vi "Main.vi"() -> ()   [LabVIEW 2021]
uses:
  <vilib>/Instr/_visa.llb/VISA Configure Serial Port (Instr).vi
  <extravilib>/ChannelInstances/Event Messenger-str/Instantiate.vi
  <extravilib>/ChannelInstances/Event Messenger-str/))Channel.vi
  <extravilib>/ChannelInstances/Event Messenger-str.lvlib
panel:
  out "Arduino":errorcluster
  in  "Exit":bool
  in  "VISA name":refnum<visa-resource-name>
  out "Ready":bool
  out "Finish":bool
  out "Start":bool
  out "Time":picture
  in  "Ready?":bool
  in  "Reset":bool
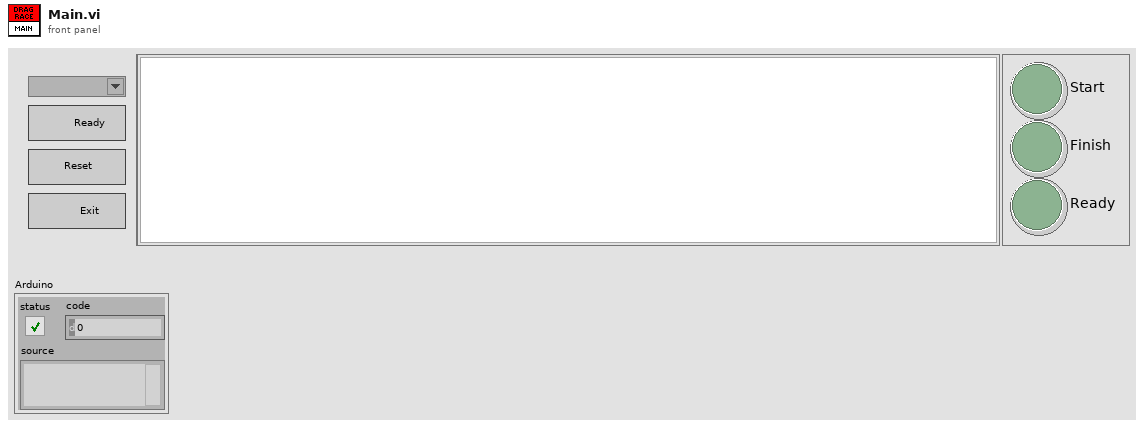
[diagram p1: front panel]
types:
  T1 = enum8{"Enabled", "Disabled", "Disabled and Grayed Out"}
  T2 = typedef "Event Messenger-str.lvlib/))Channel.ctl" = refnum<queue>
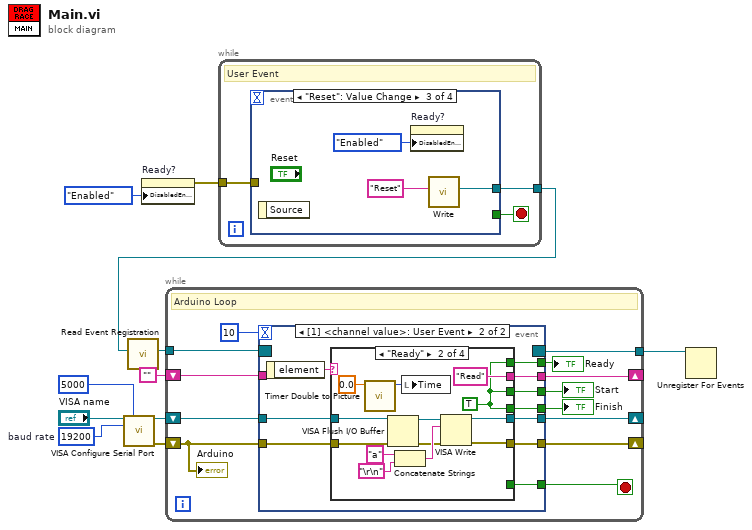
[diagram p0: block diagram]
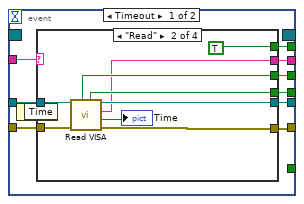
[diagram p2: hidden frame]
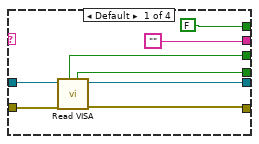
[diagram p3: hidden frame]
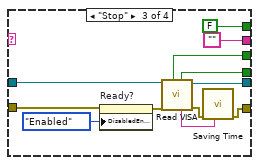
[diagram p4: hidden frame]
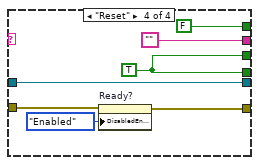
[diagram p5: hidden frame]
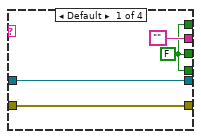
[diagram p6: hidden frame]
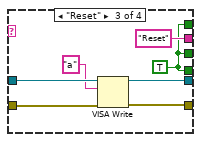
[diagram p7: hidden frame]
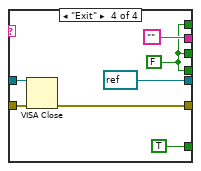
[diagram p8: hidden frame]
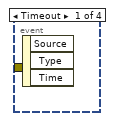
[diagram p9: hidden frame]
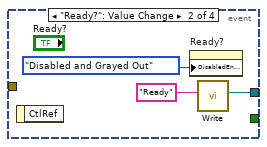
[diagram p10: hidden frame]
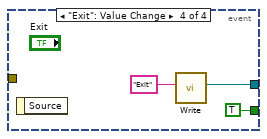
[diagram p11: hidden frame]
diagram:
  w10 = u32 19200  # baud rate
  n1 = call-poly "VISA Configure Serial Port"("VISA resource name"="VISA name", "timeout (10sec)"=u32 5000, "baud rate (9600)"=w10) -> ("VISA resource name out"=w9:refnum<visa-resource-name>, "error out"=w8:errorcluster)  [unwired: 11 in]
  n2 = property on="Ready?" class="Bool"("DisabledEnum"=T1."Enabled" ("Disabled")) -> (error out=w3:errorcluster)  [unwired: 2 in, 1 out]
  n3 = while {
    tunnel: [w14] -> w7
    tunnel: w3 -> [w12]
    stop <- w13 stop-if-true
    # "User Event"
    n4 = event shown="[2] \"Reset\": Value Change" {
      selector: _ -> [_ _ _ _]
      dyn-events: _ -> [_ _ _ _]
      timeout: _ -> [_ _ _ _]
      tunnel: [_ w16 w19 w22] -> w14
      tunnel: [_ _ _ TRUE] -> w13
      tunnel: w12 -> [_ _ _ _]
      event Timeout {
        n5 = event-data() -> ()  [unwired: 1 in, 3 out]
      }
      event "Ready?": Value Change {
        n6 = event-data() -> ()  [unwired: 1 in, 1 out]
        n7 = property on="Ready?" class="Bool"("DisabledEnum"=T1."Disabled and Grayed Out" ("Disabled")) -> ()  [unwired: 2 in, 2 out]
        n8 = call <extravilib>:"Write.vi"("element"="Ready") -> ("channel"=w16:T2)  [unwired: 9 in, 1 out]
      }
      event "Reset": Value Change {
        n9 = event-data() -> ()  [unwired: 1 in, 1 out]
        n10 = property on="Ready?" class="Bool"("DisabledEnum"=T1."Enabled" ("Disabled")) -> ()  [unwired: 2 in, 2 out]
        n11 = call <extravilib>:"Write.vi"("element"="Reset") -> ("channel"=w19:T2)  [unwired: 9 in, 1 out]
      }
      event "Exit": Value Change {
        n12 = event-data() -> ()  [unwired: 1 in, 1 out]
        n13 = call <extravilib>:"Write.vi"("element"="Exit") -> ("channel"=w22:T2)  [unwired: 9 in, 1 out]
      }
    }
  }
  n14 = call <extravilib>:"Read Event Registration.vi"("channel"=w7) -> ("event registration refnum"=w6:refnum<event-registration>)  [unwired: 10 in]
  n15 = while {
    shift-right: [w32] -> _
    shift-left: w9 -> [w34]
    shift-right: [w31] -> _
    shift-left: w8 -> [w33]
    tunnel: w6 -> [w36]
    tunnel: [w35] -> w5
    shift-right: [w29] -> _
    shift-left: "" -> [w28]
    stop <- w27 stop-if-true
    # "Arduino Loop"
    n16 = event shown="[1] <channel value>: User Event" {
      selector: w36 -> [_ _]
      dyn-events: [_ _] -> w35
      timeout: 10 -> [_ _]
      tunnel: w34 -> [w45 w90]
      tunnel: w33 -> [w44 w89]
      tunnel: [w43 w88] -> w32
      tunnel: [w42 w87] -> w31
      tunnel: [w40 w86] -> w29
      tunnel: w28 -> [w41 _]
      tunnel: [_ w85] -> w27
      tunnel: [w39 w83] -> w26
      tunnel: [w38 w84] -> w25
      tunnel: [w37 w82] -> w24
      event Timeout {
        n17 = event-data() -> ()  [unwired: 1 in, 1 out]
        n18 = case shown="\"Read\"" w41 {
          tunnel: w45 -> [w53 w60 w70 w81]
          tunnel: w44 -> [w52 w59 w73 w79]
          tunnel: [w51 w62 w69 w81] -> w43
          tunnel: [w50 w61 w64 w78] -> w42
          tunnel: [w49 w58 w67 w77] -> w38
          tunnel: [w48 w57 w66 w77] -> w39
          tunnel: [FALSE ("Ready") TRUE ("Ready") FALSE ("Ready") FALSE ("Ready")] -> w37
          tunnel: ["" w54 "" ""] -> w40
          frame Default {
            n19 = call "Read VISA.vi"("error in"=w52, "VISA Refnum in"=w53) -> ("error out"=w50:errorcluster, "VISA Refnum out"=w51:refnum<visa-resource-name>, "Finish Connect?"=w48:bool, "Start Connect?"=w49:bool)  [unwired: 3 in, 3 out]
          }
          frame "Read" {
            n20 = call "Read VISA.vi"("error in"=w59, "VISA Refnum in"=w60) -> ("error out"=w61:errorcluster, "Display Time"=→"Time":picture, "Command"=w54:string, "VISA Refnum out"=w62:refnum<visa-resource-name>, "Finish Connect?"=w57:bool, "Start Connect?"=w58:bool)  [unwired: 3 in, 1 out]
          }
          frame "Stop" {
            n21 = property on="Ready?" class="Bool"(error in=w73, "DisabledEnum"=T1."Enabled" ("Disabled")) -> (error out=w68:errorcluster)  [unwired: 1 in, 1 out]
            n22 = call "Read VISA.vi"("error in"=w68, "VISA Refnum in"=w70) -> ("error out"=w65:errorcluster, "VISA Refnum out"=w69:refnum<visa-resource-name>, "File Save Time"=w63:string, "Finish Connect?"=w66:bool, "Start Connect?"=w67:bool)  [unwired: 3 in, 2 out]
            n23 = call "Saving Time.vi"("File Save Time"=w63, "error in (no error)"=w65) -> ("error out"=w64:errorcluster)  [unwired: 9 in]
          }
          frame "Reset" {
            w77 = TRUE ("Start Connect?")
            n24 = property on="Ready?" class="Bool"(error in=w79, "DisabledEnum"=T1."Enabled" ("Disabled")) -> (error out=w78:errorcluster)  [unwired: 1 in, 1 out]
          }
        }
      }
      event User Event {
        n25 = event-data() -> ("element"=w91:string)  [unwired: 1 in]
        n26 = case shown="\"Ready\"" w91 {
          tunnel: w90 -> [w95 w97 w115 w121]
          tunnel: w89 -> [w94 w100 w114 w120]
          tunnel: [w95 w105 w113 refnum<visa-resource-name> refnum ("VISA resource name out")] -> w88
          tunnel: [w94 w104 w112 w119] -> w87
          tunnel: ["" "Read" "Reset" ""] -> w86
          tunnel: [_ _ _ TRUE] -> w85
          tunnel: [w92 w96 w109 w116] -> w84
          tunnel: [w92 w96 w109 w116] -> w83
          tunnel: [w92 w96 w109 w116] -> w82
          frame Default {
            w92 = FALSE ("Start Connect?")
          }
          frame "Ready" {
            w96 = TRUE ("Start Connect?")
            n27 = call "Timer Double to Picture.vi"("Time (sec)"=0.0) -> ("new picture"=w107:picture)  [unwired: 9 in, 1 out]
            n28 = VISA Flush I/O Buffer(VISA resource name=w97, error in (no error)=w100) -> (VISA resource name out=w99:refnum<visa-resource-name>, error out=w98:errorcluster)  [unwired: 1 in]
            n29 = Concatenate Strings("a" ("write buffer"), "\r\n") -> (w101:string)
            n30 = local write "Time"(w107) -> ()
            n31 = VISA Write(VISA resource name=w99, write buffer=w101, error in (no error)=w98) -> (VISA resource name out=w105:refnum<visa-resource-name>, error out=w104:errorcluster)  [unwired: 1 out]
          }
          frame "Reset" {
            w109 = TRUE ("Start Connect?")
            n32 = VISA Write(VISA resource name=w115, write buffer="a", error in (no error)=w114) -> (VISA resource name out=w113:refnum<visa-resource-name>, error out=w112:errorcluster)  [unwired: 1 out]
          }
          frame "Exit" {
            w116 = FALSE ("Start Connect?")
            n33 = VISA Close(VISA resource name=w121, error in (no error)=w120) -> (error out=w119:errorcluster)
          }
        }
      }
    }
    "Start" <- w25
    "Finish" <- w26
    "Ready" <- w24
    "Arduino" <- w33
  }
  n34 = Unregister For Events(event registration refnum=w5) -> ()  [unwired: 1 in, 1 out]
